vi "pii.vi"() -> ()   [LabVIEW 2023]
panel:
  out "Ajanotto":u32
  out "Hex pii":string[](array[string])
  in  "Aloituskohta":dbl
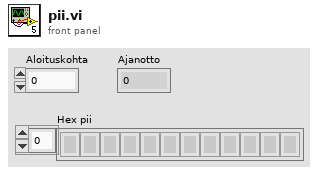
[diagram p1: front panel]
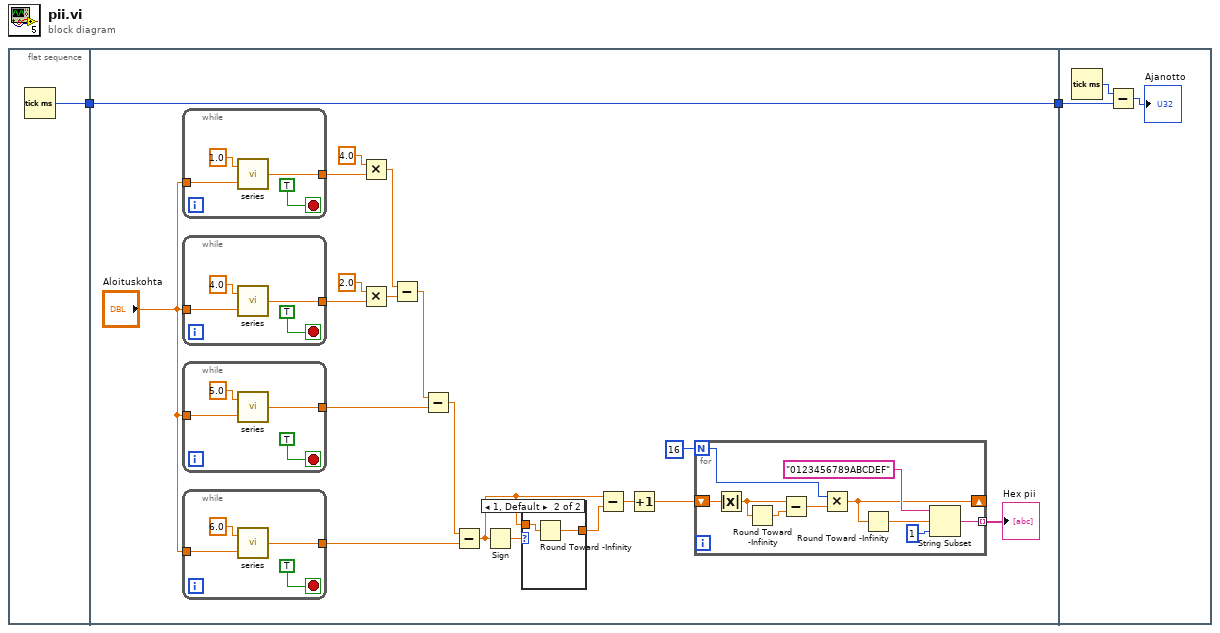
[diagram p0: block diagram]
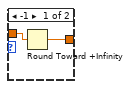
[diagram p2: hidden frame]
diagram:
  n1 = flat-sequence {
    tunnel: [w3] -> w2
    tunnel: w2 -> [w4]
    tunnel: [w4] -> w1
    tunnel: w1 -> [w53]
    frame #0 {
      n2 = Tick Count (ms)() -> (millisecond timer value=w3:u32)
    }
    frame #1 {
      n3 = while {
        tunnel: "Aloituskohta" -> [w48]
        tunnel: [w46] -> w21
        stop <- TRUE stop-if-true
        n4 = call "series.vi"("ic"=w48, "m"=1.0) -> ("s"=w46:dbl)
      }
      n5 = while {
        tunnel: "Aloituskohta" -> [w44]
        tunnel: [w42] -> w18
        stop <- TRUE stop-if-true
        n6 = call "series.vi"("ic"=w44, "m"=4.0) -> ("s"=w42:dbl)
      }
      n7 = while {
        tunnel: "Aloituskohta" -> [w40]
        tunnel: [w38] -> w14
        stop <- TRUE stop-if-true
        n8 = call "series.vi"("ic"=w40, "m"=5.0) -> ("s"=w38:dbl)
      }
      n9 = while {
        tunnel: "Aloituskohta" -> [w36]
        tunnel: [w34] -> w12
        stop <- TRUE stop-if-true
        n10 = call "series.vi"("ic"=w36, "m"=6.0) -> ("s"=w34:dbl)
      }
      n11 = Multiply(x=4.0, y=w21) -> (x*y=w17:dbl)
      n12 = Multiply(x=2.0, y=w18) -> (x*y=w16:dbl)
      n13 = Subtract(x=w17, y=w16) -> (x-y=w15:dbl)
      n14 = Subtract(x=w15, y=w14) -> (x-y=w13:dbl)
      n15 = Subtract(x=w13, y=w12) -> (x-y=w10:dbl)
      n16 = Sign(1:w10) -> (0:w11:dbl)
      n17 = case shown="1, Default" w11 {
        tunnel: w10 -> [w50 w52]
        tunnel: [w49 w51] -> w9
        frame -1 {
          n18 = Round Toward +Infinity(x=w50) -> (ceil(x): smallest int >= x=w49:dbl)
        }
        frame 1, Default {
          n19 = Round Toward -Infinity(1:w52) -> (0:w51:dbl)
        }
      }
      n20 = Subtract(x=w10, y=w9) -> (x-y=w8:dbl)
      n21 = Increment(x=w8) -> (x+1=w6:dbl)
      n22 = for {
        N: 16 -> [w27]
        shift-right: [w24] -> _
        shift-left: w6 -> [w28]
        tunnel: [w25] -> w5 mode=indexing
        n23 = Absolute Value(x=w28) -> (abs(x)=w31:dbl)
        n24 = Round Toward -Infinity(1:w31) -> (0:w30:dbl)
        n25 = Subtract(x=w31, y=w30) -> (x-y=w29:dbl)
        n26 = Multiply(x=w27, y=w29) -> (x*y=w24:dbl)
        n27 = Round Toward -Infinity(1:w24) -> (0:w23:dbl)
        n28 = String Subset(string="0123456789ABCDEF", offset (0)=w23, length (rest)=1 ("length (rest)")) -> (substring=w25:string)
      }
      "Hex pii" <- w5
    }
    frame #2 {
      n29 = Tick Count (ms)() -> (millisecond timer value=w54:u32)
      n30 = Subtract(x=w54, y=w53) -> (x-y=→"Ajanotto":u32)
    }
  }
